vi "Auto-Refresh Read.vi"(8 "error in (no error)":errorcluster, 11 "CAP-USB-1 in":refnum<class "CAP-USB-1.lvclass">) -> (0 "error out":errorcluster, 1 "Control Data":T1, 2 "1 Sample":T2, 3 "CAP-USB-1 out":refnum<class "CAP-USB-1.lvclass">)   [LabVIEW 2014, in "CAP-USB-1.lvlib" / "CAP-USB-1.lvclass"]
doc: "Realiza la lectura de los valores enviados por el equipo"
uses:
  CAP-USB-1.lvclass
  DriverMasterSync/build/DriverMasterSync.lvlibp/APIs/Data Queue/Acquisition Data 1 Sample Cluster.ctl
  DriverMasterSync/build/DriverMasterSync.lvlibp/APIs/Data Queue/Control Data Cluster.ctl
  CAP-USB-1.lvclass/CAP-USB-1.ctl
  API/CAP-USB/CAP-USB.lvlib
  DriverMasterSync/build/DriverMasterSync.lvlibp/Modules/HAL/DriverMasterSync/DriverMasterSyncClass/DriverMasterSync.lvclass
  DriverMasterSync/build/DriverMasterSync.lvlibp/APIs/Data Queue/WINFAS 2 Data Queue.lvlib
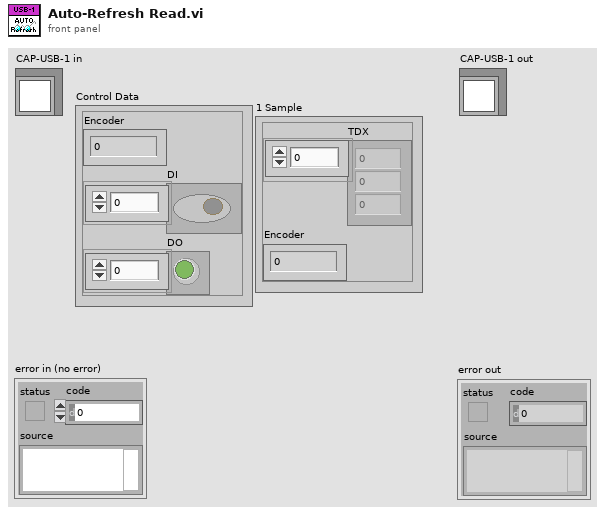
[diagram p1: front panel]
types:
  T1 = typedef "DriverMasterSync.lvlibp/WINFAS 2 Data Queue.lvlib/Control Data Cluster.ctl" = cluster{"Encoder":sgl, "DI":bool[], "DO":bool[]}
  T2 = typedef "DriverMasterSync.lvlibp/WINFAS 2 Data Queue.lvlib/Acquisition Data 1 Sample Cluster.ctl" = cluster{"TDX":sgl[], "Encoder":sgl}
  T3 = typedef "DriverMasterSync.lvlibp/WINFAS 2 Data Queue.lvlib/Acquisition Data Cluster.ctl" = T2[]
  T4 = cluster{"Entradas":bool[], "Salidas":bool[], "Valor Encoder":u16, "Valor Transductores":u16[], "Orden Transd":u32[]}[]
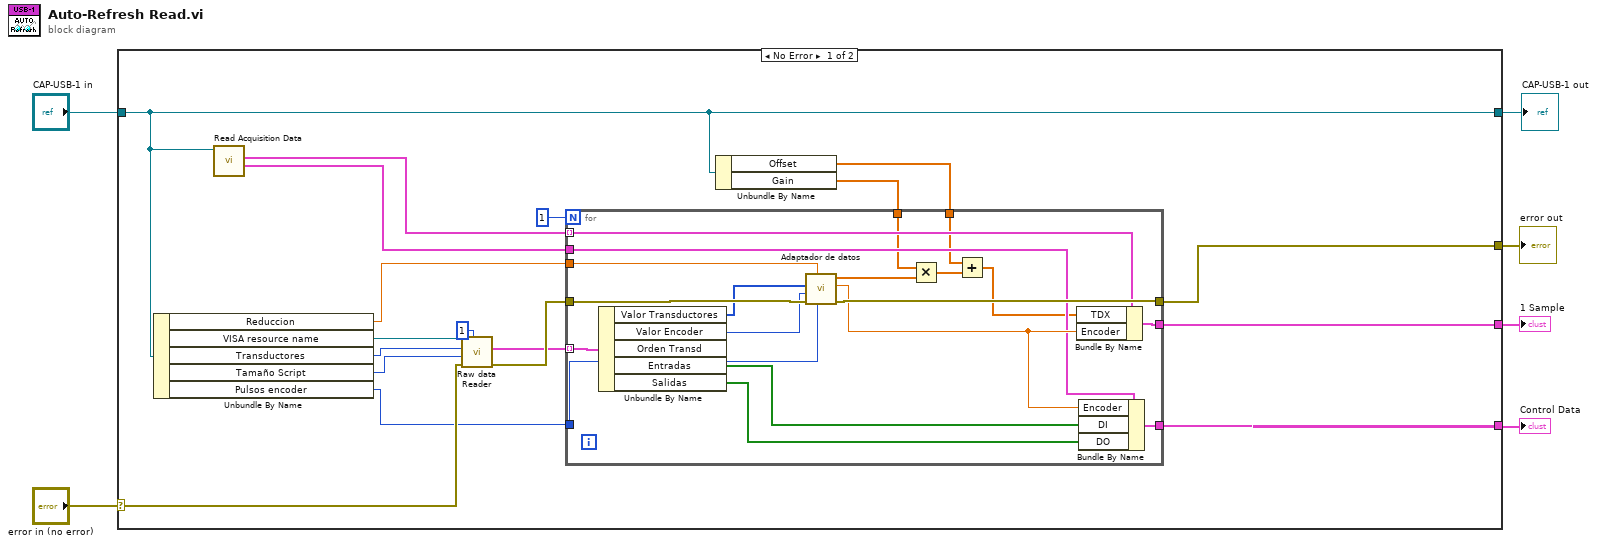
[diagram p0: block diagram]
diagram:
  n1 = case shown="No Error" "error in (no error)" {
    selector: "error in (no error)" -> [w21 w45]
    tunnel: [w10 w45] -> w5
    tunnel: [w9 w44] -> w3
    tunnel: "CAP-USB-1 in" -> [w9 w44]
    tunnel: [w11 _] -> w2
    tunnel: [w15 _] -> w1
    frame No Error {
      n2 = Unbundle By Name(w9) -> ("Reduccion"=w12:sgl, "VISA resource name"=w19:refnum<visa-resource-name>, "Transductores"=w24:u64, "Tamaño Script"=w23:i32, "Pulsos encoder"=w17:u16)
      n3 = call "Read Acquisition Data.vi"("DriverMasterSync in"=w9) -> ("Control Data"=w16:T1, "Acquisition Data"=w20:T3)  [unwired: 7 in, 2 out]
      n4 = call "Raw data Reader.vi"("Num de tramas"=u32 1, "error in (no error)"=w21, "Tamaño Script"=w23, "TRANSDUCTORES"=w24, "VISA Refnum in"=w19) -> ("error out"=w18:errorcluster, "Raw data"=w14:T4)  [unwired: 2 in, 1 out]
      n5 = Unbundle By Name(w9) -> ("Offset"=w7:sgl[], "Gain"=w8:sgl[])
      n6 = for {
        N: 1 -> [_]
        tunnel: w20 -> [w30] mode=indexing
        tunnel: w14 -> [w43] mode=indexing
        tunnel: [w42] -> w11
        tunnel: w18 -> [w41]
        tunnel: [w34] -> w10
        tunnel: w17 -> [w39]
        tunnel: w16 -> [w31]
        tunnel: [w36] -> w15
        tunnel: w12 -> [w32]
        tunnel: w8 -> [w29]
        tunnel: w7 -> [w26]
        n7 = Unbundle By Name(w43) -> ("Valor Transductores"=w40:u16[], "Valor Encoder"=w35:u16, "Entradas"=w38:bool[], "Salidas"=w37:bool[])  [unwired: 1 out]
        n8 = call "Adaptador de datos.vi"("Cant. de pulsos"=w39, "Reduccion"=w32, "error in (no error)"=w41, "Encoder"=w35, "Transductores"=w40) -> ("error out"=w34:errorcluster, "Encoder"=w33:sgl, "Transductores"=w28:sgl[])  [unwired: 4 in]
        n9 = Multiply(x=w29, y=w28) -> (x*y=w27:sgl[])
        n10 = Add(x=w26, y=w27) -> (x+y=w25:sgl[])
        n11 = Bundle By Name(cluster=w30, "TDX"=w25, "Encoder"=w33) -> (w42:T2)
        n12 = Bundle By Name(cluster=w31, "Encoder"=w33, "DI"=w38, "DO"=w37) -> (w36:T1)
      }
    }
    frame Error {
    }
  }
  "error out" <- w5
  "CAP-USB-1 out" <- w3
  "1 Sample" <- w2
  "Control Data" <- w1
